vi "GEA3 PID Parameters.vi"() -> ()   [LabVIEW 2020]
uses:
  type defs/ERD Write Data In.ctl
  type defs/Data Type.ctl
  type defs/Data In.ctl
  library/GEA2_Toolkit.lvlib
panel:
  out "Conv Message Out":string
  out "GEA Message":T1 {"Command" format="%02x"; "Destination" format="%02x"; "Source" format="%02x"}
  in  "ERD Write Data In":T2={"ERD Number"=61460, "Data Type"=enum."string", "Data"=""} {"ERD Number" format="%.0x"}
  in  "Kp Qbits Value":i32
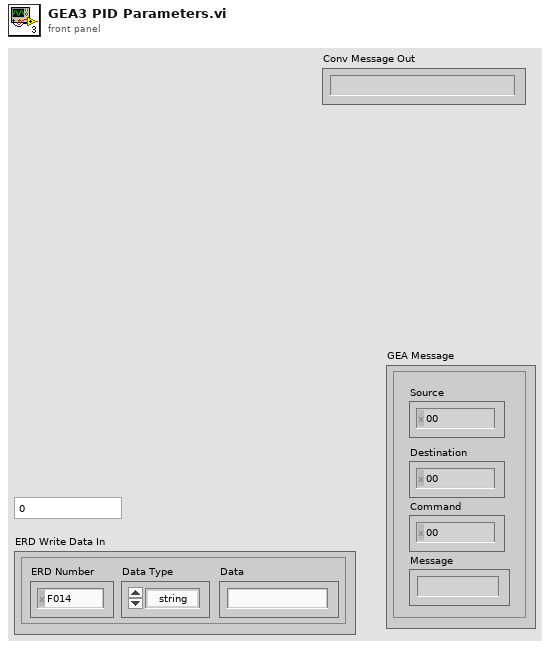
[diagram p1: front panel]
types:
  T1 = typedef "GEA2_Toolkit.lvlib/Data In.ctl" = cluster{"Source":u8, "Destination":u8, "Command":u8, "Message":string}
  T2 = typedef "GEA2_Toolkit.lvlib/ERD Write Data In.ctl" = cluster{"ERD Number":u16, "Data Type":T3, "Data":string}
  T3 = typedef "GEA2_Toolkit.lvlib/Data Type.ctl" = enum16{"string", "boolean", "uint8_t", "uint16_t", "uint32_t", "uint64_t", "int8_t", "int16_t", "int32_t", "int64_t"}
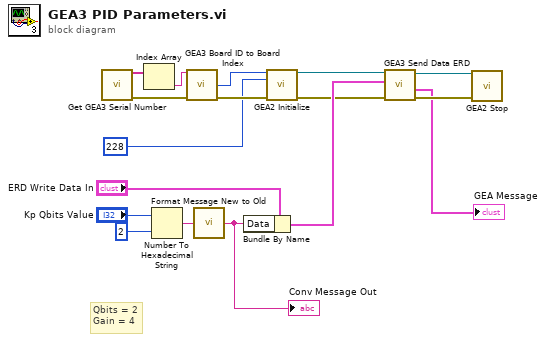
[diagram p0: block diagram]
diagram:
  # "Qbits = 2\nGain = 4"
  n1 = call "Get GEA3 Serial Number.vi"() -> ("GEA3 Serial Numbers"=w14:string[], "Error Out"=w15:errorcluster)  [unwired: 14 in]
  n2 = Index Array(array=w14) -> (element=w13:string)  [unwired: 1 in]
  n3 = Number To Hexadecimal String(1:i16 2 ("width (-)"), 2:"Kp Qbits Value") -> (0:w11:string)
  n4 = call "GEA3 Board ID to Board Index.vi"("GEA3 Serial Number"=w13, "Error In"=w15) -> ("Board Index"=w16:i32, "Error Out"=w17:errorcluster)  [unwired: 9 in, 3 out]
  n5 = call "Format Message New to Old.vi"("Raw Message In"=w11) -> ("Conv Message Out"=w2:string)  [unwired: 14 in]
  "Conv Message Out" <- w2
  n6 = Bundle By Name(cluster="ERD Write Data In", "Data"=w2) -> (w7:T2)
  n7 = call "GEA2 Initialize.vi"("Board Index"=w16, "Source Address"=u8 228, "error in"=w17) -> ("GEA2 Reference Out"=w6:refnum<k24>, "error out"=w5:errorcluster)  [unwired: 10 in, 1 out]
  n8 = call "GEA3 Send Data ERD.vi"("error in (no error)"=w5, "ERD Write Data In"=w7, ".NET Refnum in"=w6) -> ("error out"=w3:errorcluster, "GEA Message"=→"GEA Message":T1, "GEA2 Reference Out"=w4:refnum<k24>)  [unwired: 5 in, 1 out]
  n9 = call "GEA2 Stop.vi"("GEA2 Reference In"=w4, "Error In"=w3) -> ()  [unwired: 13 in, 1 out]
